vi "main_break_signal.vi"(11 "Keep Running?":bool) -> (3 "Break Notifier":refnum<notifier>)   [LabVIEW 2019]
panel:
  # "*******************************************************************\nBiogas Plant Control\n\nAuthor: Paul Zügel\nGCSC-Frankfurt am Main 2020\n\n*******************************************************************"
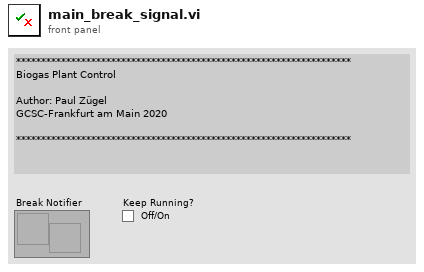
[diagram p1: front panel]
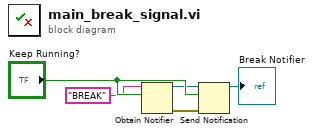
[diagram p0: block diagram]
diagram:
  n1 = Obtain Notifier(name (unnamed)="BREAK", notification data type="Keep Running?") -> (notifier out=w3:refnum<notifier>, error out=w4:errorcluster)  [unwired: 2 in, 1 out]
  n2 = Send Notification(notification="Keep Running?", notifier=w3, error in (no error)=w4) -> (notifier out=→"Break Notifier":refnum<notifier>)  [unwired: 1 out]
